vi "Read PV Type.vi"(8 "error in (no error)":errorcluster, 11 "PV in":refnum<class "PV.lvclass">) -> (0 "error out":errorcluster, 2 "PV Type":T1, 3 "PV out":refnum<class "PV.lvclass">)   [LabVIEW 2016, in "CS++ProcessVariables.lvlib" / "PV.lvclass"]
doc: "Read PV-Type from attribute."
uses:
  PV.lvclass
  PV Type.ctl
  PV.lvclass/PV.ctl
  CS++ProcessVariables.lvlib
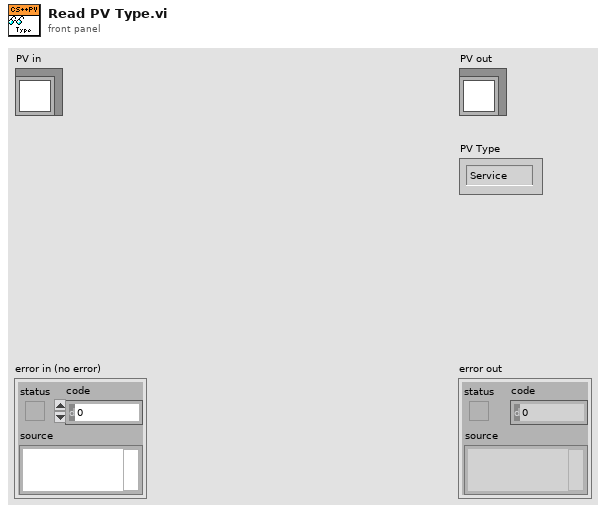
[diagram p1: front panel]
types:
  T1 = typedef "CS++ProcessVariables.lvlib/PV Type.ctl" = enum16{"Service", "Command"}
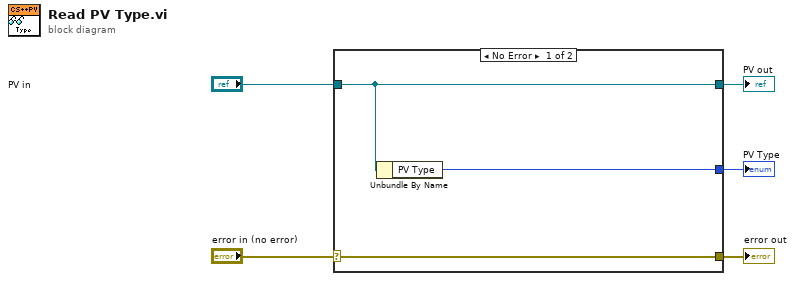
[diagram p0: block diagram]
diagram:
  n1 = case shown="No Error" "error in (no error)" {
    selector: "error in (no error)" -> [w8 w9]
    tunnel: [w8 w9] -> w4
    tunnel: [w7 w10] -> w2
    tunnel: "PV in" -> [w7 w10]
    tunnel: [w6 _] -> w1
    frame No Error {
      n2 = Unbundle By Name(w7) -> ("PV Type"=w6:T1)
    }
    frame Error {
    }
  }
  "error out" <- w4
  "PV out" <- w2
  "PV Type" <- w1
